vi "List - Get Selected Value.vi"(6 "Select":enum16{"All", "True", "False"}(ring), 8 "Error In":errorcluster, 11 "List In":cluster{"Name":string, "Selected":bool}[](array[cluster])) -> (0 "Error Out":errorcluster, 3 "List Out":string[](array[string]))   [LabVIEW 2020]
doc: "This VI use to update selected value."
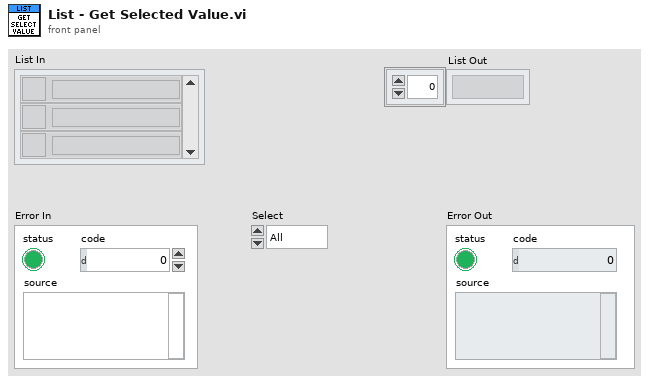
[diagram p1: front panel]
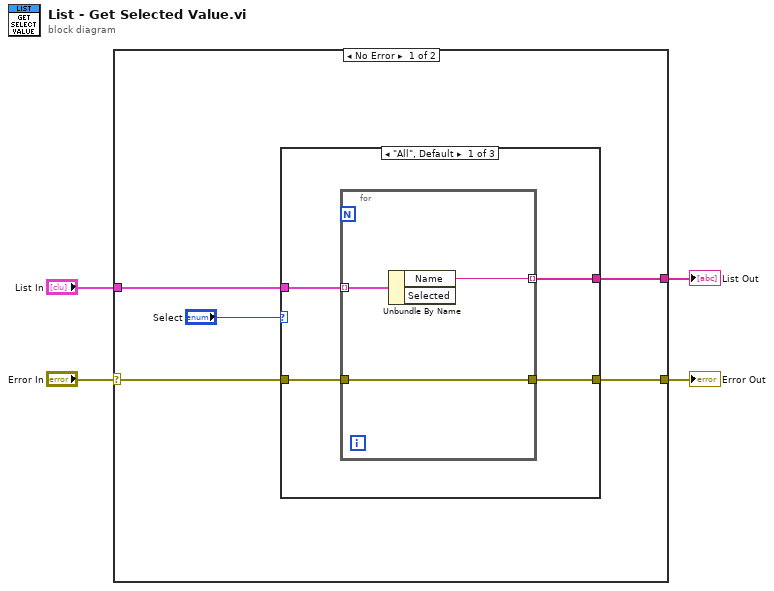
[diagram p0: block diagram]
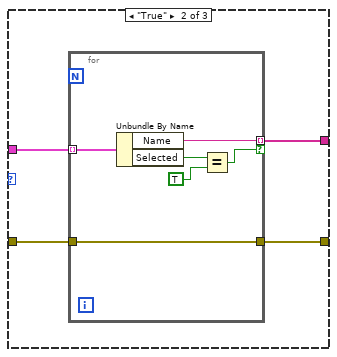
[diagram p2: hidden frame]
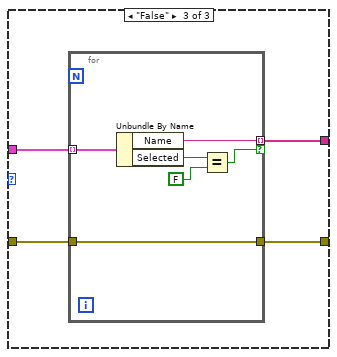
[diagram p3: hidden frame]
diagram:
  n1 = case shown="No Error" "Error In" {
    selector: "Error In" -> [w9 w38]
    tunnel: [w8 w38] -> w3
    tunnel: "List In" -> [w7 _]
    tunnel: [w6 string[] []] -> w1
    frame No Error {
      n2 = case shown="\"All\", Default" "Select" {
        tunnel: w9 -> [w13 w20 w30]
        tunnel: [w12 w19 w29] -> w8
        tunnel: w7 -> [w11 w18 w28]
        tunnel: [w10 w17 w27] -> w6
        frame "All", Default {
          n3 = for {
            tunnel: w11 -> [w15] mode=indexing
            tunnel: [w16] -> w12
            tunnel: w13 -> [w16]
            tunnel: [w14] -> w10 mode=indexing
            n4 = Unbundle By Name(w15) -> ("Name"=w14:string)  [unwired: 1 out]
          }
        }
        frame "True" {
          n5 = for {
            tunnel: w18 -> [w25] mode=indexing
            tunnel: [w26] -> w19
            tunnel: w20 -> [w26]
            tunnel: [w24] -> w17 mode=indexing if=w22
            n6 = Unbundle By Name(w25) -> ("Name"=w24:string, "Selected"=w23:bool)
            n7 = Equal?(x=w23, y=TRUE) -> (x = y?=w22:bool)
          }
        }
        frame "False" {
          n8 = for {
            tunnel: w28 -> [w35] mode=indexing
            tunnel: [w36] -> w29
            tunnel: w30 -> [w36]
            tunnel: [w34] -> w27 mode=indexing if=w32
            n9 = Unbundle By Name(w35) -> ("Name"=w34:string, "Selected"=w33:bool)
            n10 = Equal?(x=w33, y=FALSE) -> (x = y?=w32:bool)
          }
        }
      }
    }
    frame Error {
    }
  }
  "Error Out" <- w3
  "List Out" <- w1
